vi "Set Translation.vi"(8 "error in (no error)":errorcluster, 10 "Translation":cluster{"X":sgl, "Y":sgl, "Z":sgl}, 11 "Scene Object":refnum<vi>) -> (0 "error out":errorcluster, 3 "Translated Object":refnum<vi>)   [LabVIEW 2017, in "NI_3D Picture Control.lvlib"]
doc: "Clears any translations previously applied to an object in a 3D scene and translates the object by the vector you specify. This VI performs an absolute translation from the object's initial position."
uses:
  <vilib>/picture/3D Picture Control/NI_3D Picture Control.lvlib
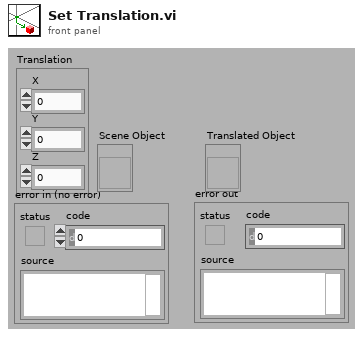
[diagram p1: front panel]
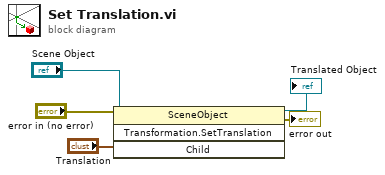
[diagram p0: block diagram]
diagram:
  n1 = invoke class="SceneObject" method="Transformation.SetTranslation"(reference="Scene Object", error in="error in (no error)", "Child"="Translation") -> (reference out=→"Translated Object":refnum<vi>, error out=→"error out":errorcluster)  [unwired: 1 in, 2 out]
